vi "To 2D Bool Tree Data.vi"(10 "2D Bool":bool[][](array[boolean])) -> (3 "2D Bool Tree Data":refnum<class "2D Bool.lvclass">)   [LabVIEW 2017, in "Tree API.lvlib" / "2D Bool.lvclass"]
doc: "Convert a 2D Bool value to Tree Data type."
uses:
  2D Bool.lvclass
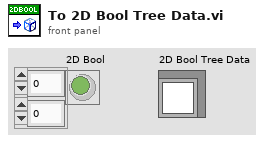
[diagram p1: front panel]
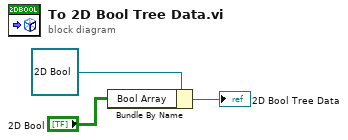
[diagram p0: block diagram]
diagram:
  n1 = Bundle By Name(cluster=refnum<class "2D Bool.lvclass"> refnum ("Tree API.lvlib:2D Bool.lvclass"), "Bool Array"="2D Bool") -> (→"2D Bool Tree Data":refnum<class "2D Bool.lvclass">)
